vi "Measure Power Calibration Data.vi"(7 "Channel (1)":i32=1, 8 "error in (no error)":errorcluster, 9 "Port 1 (1)":i32=1, 10 "Power Sensor (0:Power Sensor A)":u16(ring) items=["Power Sensor A", "Power Sensor B"], 11 "VISA resource name":refnum<visa-resource-name>) -> (0 "error out":errorcluster, 3 "VISA resource name out":refnum<visa-resource-name>)   [LabVIEW 2011, in "Agilent ENA Series.lvlib"]
doc: "For selected port, measure the power calibration data using the specified power sensor. When the measurement is complete successfully, the power level error correction is automatically enabled."
uses:
  Agilent ENA Series.lvlib
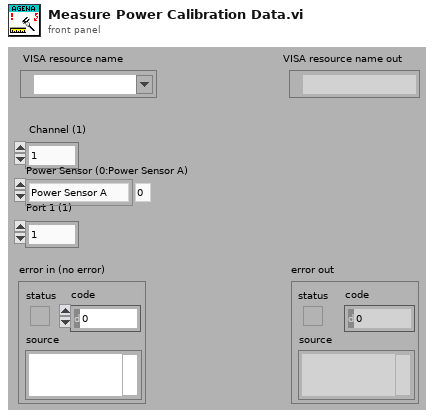
[diagram p1: front panel]
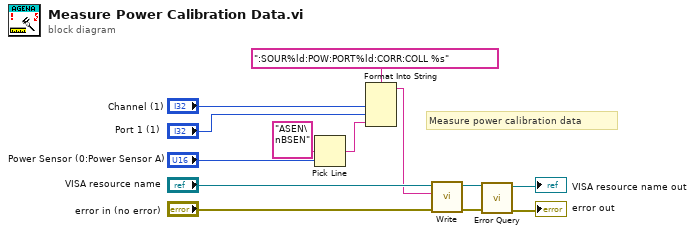
[diagram p0: block diagram]
diagram:
  # "Measure power calibration data"
  n1 = Pick Line(multi-line string="ASEN\nBSEN", line index="Power Sensor (0:Power Sensor A)") -> (output string=w8:string)  [unwired: 1 in]
  n2 = Format Into String(format string=":SOUR%ld:POW:PORT%ld:CORR:COLL %s", "Channel (1)", "Port 1 (1)", w8) -> (resulting string=w7:string)  [unwired: 2 in, 1 out]
  n3 = call "Write.vi"("error in (no error)"="error in (no error)", "String ()"=w7, "VISA resource name"="VISA resource name") -> ("error out"=w3:errorcluster, "VISA resource name out"=w4:refnum<visa-resource-name>)  [unwired: 6 in, 1 out]
  n4 = call "Error Query.vi"("error in (no error)"=w3, "VISA resource name"=w4) -> ("error out"=→"error out":errorcluster, "VISA resource name out"=→"VISA resource name out":refnum<visa-resource-name>)  [unwired: 6 in, 2 out]
